vi "AutonomousComboBox.vi"(11 "ComboBox in":refnum<vi>) -> ()   [LabVIEW 2015]
uses:
  <vilib>/Rock Robotics/Network Tables/NT Read String Array.vi
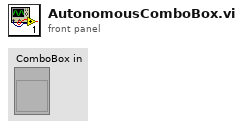
[diagram p1: front panel]
types:
  T1 = typedef "LVComboBoxStrsAndValuesArrayTypeDef.ctl" = cluster{"String":string, "Value":string}[]
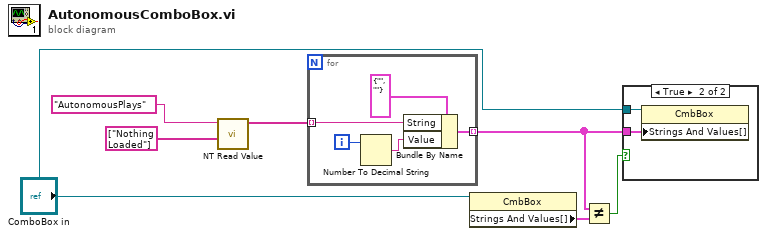
[diagram p0: block diagram]
diagram:
  n1 = call-poly <vilib>:"NT Read Value.vi"("Default Value"=string[] ["Nothing Loaded"], "Name"="AutonomousPlays") -> ("String Array"=w6:string[])  [unwired: 8 in, 1 out]
  n2 = for {
    tunnel: w6 -> [w9] mode=indexing
    tunnel: [w8] -> w7 mode=indexing
    i -> [w12]
    n3 = Number To Decimal String(number=w12) -> (decimal integer string=w11:string)  [unwired: 1 in]
    n4 = Bundle By Name(cluster=cluster{"String":string, "Value":string} {"String"="", "Value"=""}, "String"=w9, "Value"=w11) -> (w8:cluster{"String":string, "Value":string})
  }
  n5 = property on="Property Node" class="CmbBox"(reference="ComboBox in") -> ("Strings And Values[]"=w5:T1)  [unwired: 1 in, 2 out]
  n6 = Not Equal?(x=w7, y=w5) -> (x != y?=w3:bool)
  n7 = case shown="True" w3 {
    tunnel: w7 -> [_ w14]
    tunnel: "ComboBox in" -> [_ w13]
    frame False {
    }
    frame True {
      n8 = property on="Property Node" class="CmbBox"(reference=w13, "Strings And Values[]"=w14) -> ()  [unwired: 1 in, 2 out]
    }
  }
